vi "Speed to power.vi"(10 "desired velocity":dbl) -> (2 "Out power":dbl)   [LabVIEW 2017]
uses:
  Robot Global Data.vi
panel:
  out "speed?":dbl
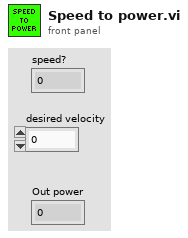
[diagram p1: front panel]
types:
  T1 = typedef "WPI_EncoderDevRef.ctl" = cluster{"DevStatus":errorcluster, "EncoderIndex":T2, "CounterIndex":T3, "DistancePerCount":dbl, "Decoding Type":T4}
  T2 = typedef "FPGA_EncoderIdx.ctl" = enum8{"Enc 0", "Enc 1", "Enc 2", "Enc 3", "Enc 4", "Enc 5", "Enc 6", "Enc 7", "Invalid"}
  T3 = typedef "FPGA_CounterCtrSystemIndex.ctl" = enum8{"Ctr 0", "Ctr 1", "Ctr 2", "Ctr 3", "Ctr 4", "Ctr 5", "Ctr 6", "Ctr 7", "Invalid"}
  T4 = typedef "WPI_EncoderType.ctl" = enum16{"1x", "2x", "4x"}
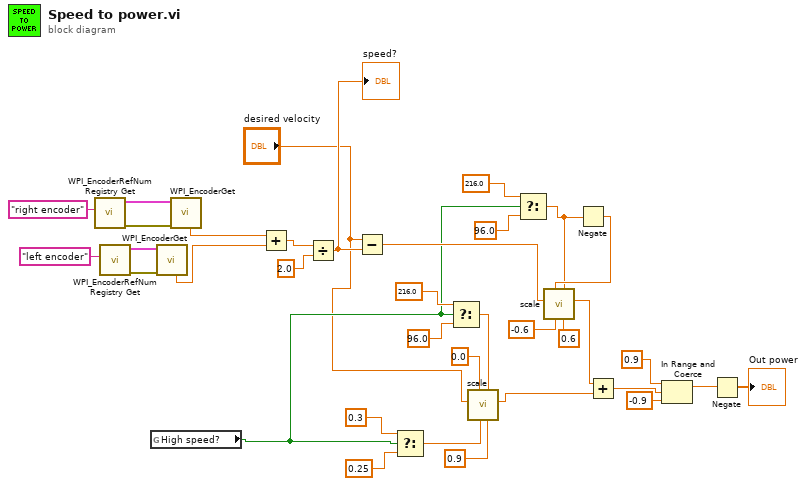
[diagram p0: block diagram]
diagram:
  n1 = call <vilib>:"WPI_EncoderRefNum Registry Get.vi"("refnum name"="right encoder") -> ("error out"=w32:errorcluster, "EncoderDevRef"=w33:T1)  [unwired: 9 in]
  n2 = call <vilib>:"WPI_EncoderRefNum Registry Get.vi"("refnum name"="left encoder") -> ("error out"=w35:errorcluster, "EncoderDevRef"=w34:T1)  [unwired: 9 in]
  n3 = global read "Robot Global Data.vi" "High speed?"() -> (w3:bool)
  n4 = call <vilib>:"WPI_EncoderGet.vi"("error in (no error)"=w35, "EncoderDevRef"=w34) -> ("Rate"=w26:dbl)  [unwired: 4 in, 5 out]
  n5 = call <vilib>:"WPI_EncoderGet.vi"("error in (no error)"=w32, "EncoderDevRef"=w33) -> ("Rate"=w27:dbl)  [unwired: 4 in, 5 out]
  n6 = Add(x=w27, y=w26) -> (x+y=w29:dbl)
  n7 = Divide(x=w29, y=2.0) -> (x/y=w2:dbl)
  "speed?" <- w2
  n8 = Subtract(x="desired velocity", y=w2) -> (x-y=w16:dbl)
  n9 = Select(t=0.3, s=w3, f=0.25) -> (s? t:f=w22:dbl)
  n10 = Select(t=216.0, s=w3, f=96.0) -> (s? t:f=w21:dbl)
  n11 = call "scale.vi"("Max"=0.9, "High"=w21, "Min"=w22, "Low"=0.0, "In Signal"="desired velocity") -> ("Output signal"=w17:dbl)  [unwired: 6 in]
  n12 = Select(t=216.0, s=w3, f=96.0) -> (s? t:f=w4:dbl)
  n13 = Negate(x=w4) -> (-x=w5:dbl)
  n14 = call "scale.vi"("Max"=0.6, "High"=w4, "Min"=-0.6, "Low"=w5, "In Signal"=w16) -> ("Output signal"=w15:dbl)  [unwired: 6 in]
  n15 = Add(x=w15, y=w17) -> (x+y=w14:dbl)
  n16 = In Range and Coerce(upper limit=0.9, x=w14, lower limit=-0.9) -> (coerced(x)=w10:dbl)  [unwired: 1 out]
  n17 = Negate(x=w10) -> (-x=→"Out power":dbl)
